vi "Slit_allow_move.vi"(1 "Translation Mode":T1=enum."Uninitialized", 2 "Rotation Mode":T1) -> (0 "Allow Move?":bool)   [LabVIEW 2015]
uses:
  SystemUtil/MotorStates.ctl
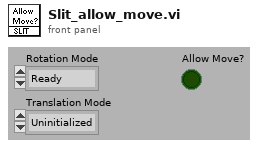
[diagram p1: front panel]
types:
  T1 = typedef "MotorStates.ctl" = enum16{"Ready", "Moving", "Uninitialized", "Error"}
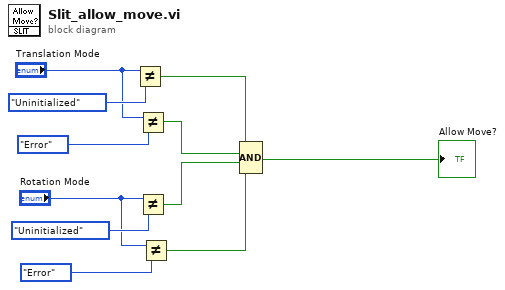
[diagram p0: block diagram]
diagram:
  n1 = Not Equal?(x="Translation Mode", y=MotorStates."Uninitialized") -> (x != y?=w5:bool)
  n2 = Not Equal?(x="Translation Mode", y=MotorStates."Error") -> (x != y?=w4:bool)
  n3 = Not Equal?(x="Rotation Mode", y=MotorStates."Uninitialized") -> (x != y?=w3:bool)
  n4 = Not Equal?(x="Rotation Mode", y=MotorStates."Error") -> (x != y?=w2:bool)
  n5 = Compound Arithmetic op=AND(w5, w4, w3, w2) -> (→"Allow Move?":bool)
